vi "字符串至布尔数组.vi"() -> ()   [LabVIEW 2022 SP3]
doc: "本VI是为《我和LabVIEW》一书编写的示例。\n关于本书的介绍请参考网页：\nhttp://ruanqizhen.spaces.live.com/blog/cns!5852D4F797C53FB6!4310.entry"
panel:
  in  "停止":bool
  out "布尔数组":bool[](array[boolean])
  in  "字符串":string
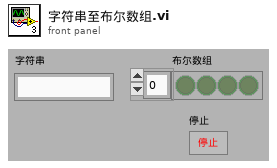
[diagram p1: front panel]
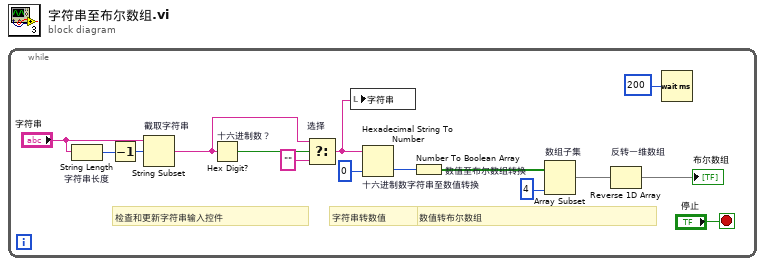
[diagram p0: block diagram]
diagram:
  n1 = while {
    stop <- "停止" stop-if-true
    # "数值转布尔数组"
    # "字符串转数值"
    # "检查和更新字符串输入控件"
    n2 = String Length "字符串长度"(string="字符串") -> (length=w2:i32)
    n3 = Decrement(x=w2) -> (x-1=w1:i32)
    n4 = String Subset "截取字符串"(string="字符串", offset (0)=w1) -> (substring=w14:string)  [unwired: 1 out]
    n5 = Hex Digit? "十六进制数？"(1:w14) -> (0:w15:bool)
    n6 = Select "选择"(t=w14, s=w15, f="") -> (s? t:f=w12:string)
    n7 = local write "字符串"(w12) -> ()
    n8 = Hexadecimal String To Number "十六进制数字符串至数值转换"(string=w12, default (0uL)=u8 0 ("默认(0 U32)")) -> (number=w10:u8)  [unwired: 2 out]
    n9 = Number To Boolean Array "数值至布尔数组转换"(number=w10) -> (Boolean array=w7:bool[])
    n10 = Array Subset "数组子集"(array=w7, length=4 ("长度")) -> (w5:bool[])  [unwired: 1 in]
    n11 = Reverse 1D Array "反转一维数组"(array=w5) -> (reversed array=→"布尔数组":bool[])
    n12 = Wait (ms)(milliseconds to wait=u32 200 ("等待时间（毫秒）")) -> ()  [unwired: 1 out]
  }
